vi "TwGetH5Descriptor.vi"(2 "TwH5Desc in":T1, 3 "filename":string, 4 "error in (no error)":errorcluster) -> (0 "TwH5Desc out":T1, 1 "error out":errorcluster)   [LabVIEW 2009]
uses:
  TwH5Dll.dll
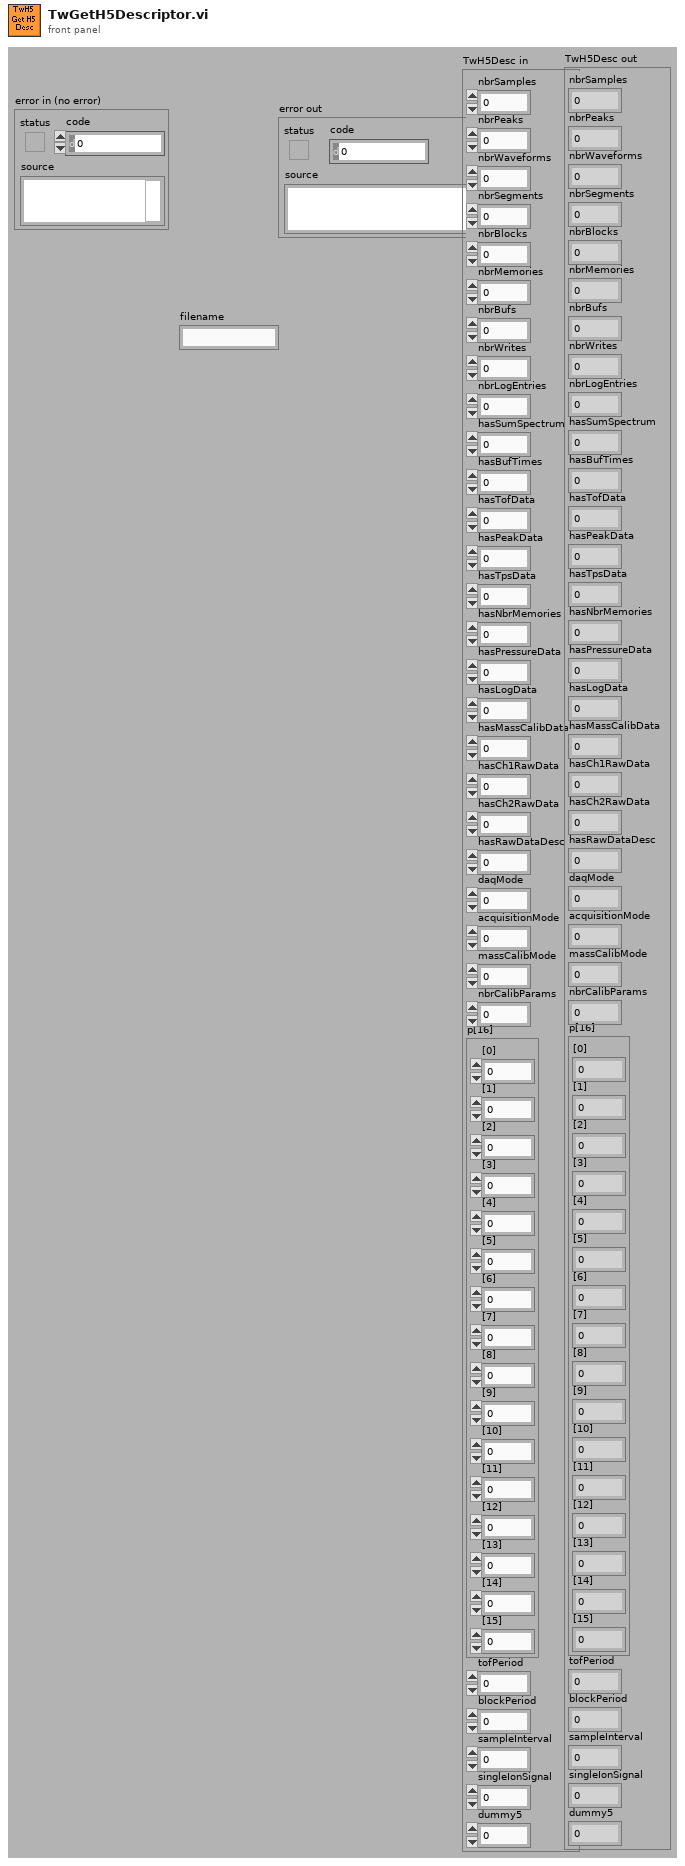
[diagram p1: front panel]
types:
  T1 = cluster{"nbrSamples":i32, "nbrPeaks":i32, "nbrWaveforms":i32, "nbrSegments":i32, "nbrBlocks":i32, "nbrMemories":i32, "nbrBufs":i32, "nbrWrites":i32, "nbrLogEntries":i32, "hasSumSpectrum":u8, "hasBufTimes":u8, "hasTofData":u8, "hasPeakData":u8, "hasTpsData":u8, "hasNbrMemories":u8, "hasPressureData":u8, "hasLogData":u8, "hasMassCalibData":u8, "hasCh1RawData":u8, "hasCh2RawData":u8, "hasRawDataDesc":u8, "daqMode":i32, "acquisitionMode":i32, "massCalibMode":i32, "nbrCalibParams":i32, "p[16]":cluster{"[0]":dbl, "[1]":dbl, "[2]":dbl, "[3]":dbl, "[4]":dbl, "[5]":dbl, "[6]":dbl, "[7]":dbl, "[8]":dbl, "[9]":dbl, "[10]":dbl, "[11]":dbl, "[12]":dbl, "[13]":dbl, "[14]":dbl, "[15]":dbl}, "tofPeriod":dbl, "blockPeriod":dbl, "sampleInterval":sgl, "singleIonSignal":sgl, "dummy5":i32}
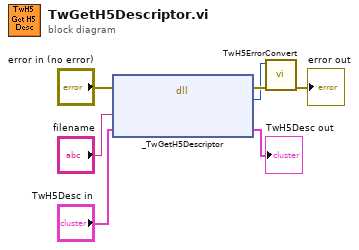
[diagram p0: block diagram]
diagram:
  n1 = dll-call lib="C:/src/85_TofDaq_current/DllWrappers/LabView/TwH5Dll/TwH5Dll.dll" fn="_TwGetH5Descriptor"(error in="error in (no error)", "filename"="filename", "descriptor"="TwH5Desc in") -> (error out=w6:errorcluster, "TwRetVal"=w5:i32, "descriptor"=→"TwH5Desc out":T1)  [unwired: 3 in, 1 out]
  n2 = call "TwH5ErrorConvert.vi"("error in (no error)"=w6, "error code"=w5) -> ("error out"=→"error out":errorcluster)  [unwired: 9 out]
